vi "PicoScopeospaPowerDetails.vi"(7 "Function":i32, 9 "PICO_USB_POWER_DETAILS In":u8[](array[numeric]), 10 "PICO_USB_POWER_DETAILS Input":T1) -> (1 "PICO_USB_POWER_DETAILS":T1 {"dataPort_"."currentPdo_" format="%x"; "dataPort_"."currentRdo_" format="%x"; "powerport_"."currentPdo_" format="%x"; "powerport_"."currentRdo_" format="%x"}, 2 "PICO_USB_POWER_DETAILS Out":u8[](array[numeric]))   [LabVIEW 2010]
doc: "This is a helper VI to read the C cluster PICO_USB_POWER_DETAILS.\nIt has two functions, controlled via input terminal \"Function\"-\n0 - (default) Outputs U8 array generated from the input cluster.\n1 - Outputs a cluster with data in the from a U8 array input terminal."
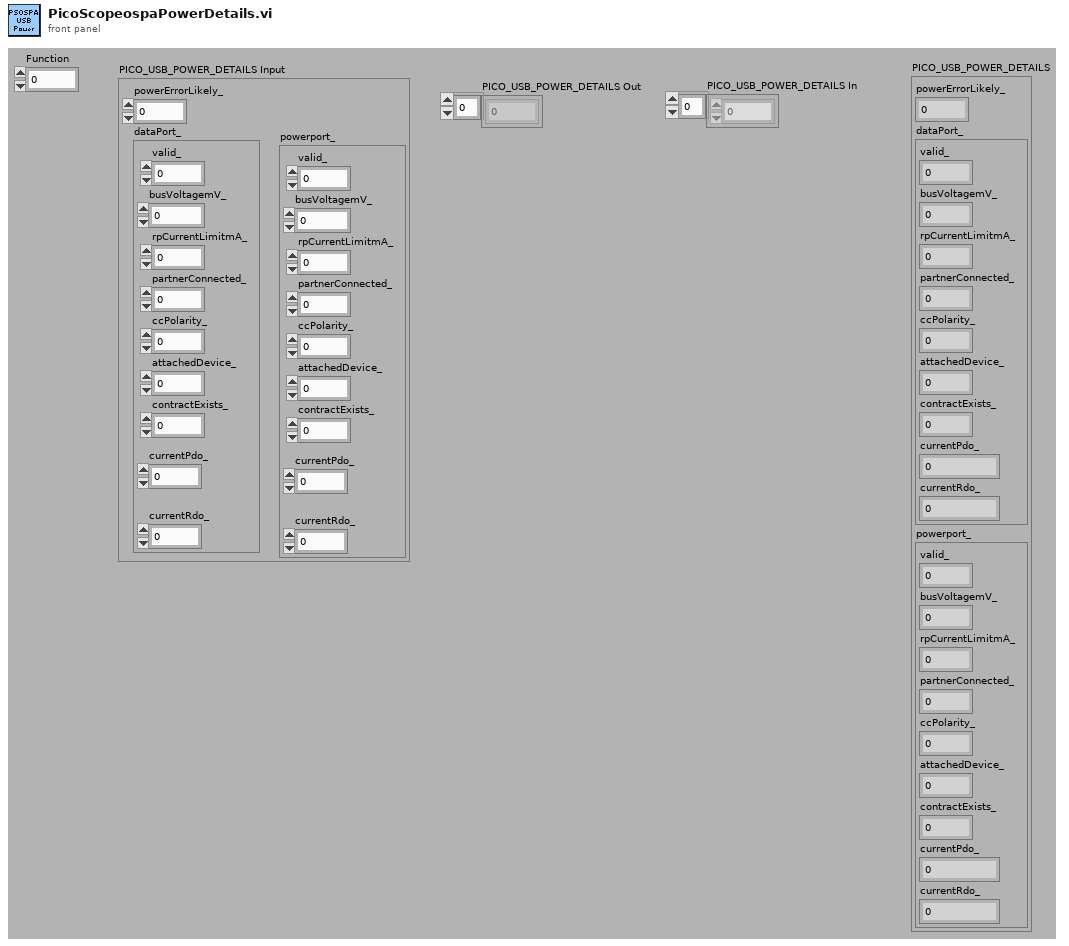
[diagram p1: front panel]
types:
  T1 = cluster{"powerErrorLikely_":u8, "dataPort_":cluster{"valid_":u8, "busVoltagemV_":u32, "rpCurrentLimitmA_":u32, "partnerConnected_":u8, "ccPolarity_":u8, "attachedDevice_":u32, "contractExists_":u8, "currentPdo_":u32, "currentRdo_":u32}, "powerport_":cluster{"valid_":u8, "busVoltagemV_":u32, "rpCurrentLimitmA_":u32, "partnerConnected_":u8, "ccPolarity_":u8, "attachedDevice_":u32, "contractExists_":u8, "currentPdo_":u32, "currentRdo_":u32}}
  T2 = cluster{"valid_":u8, "busVoltagemV_":u32, "rpCurrentLimitmA_":u32, "partnerConnected_":u8, "ccPolarity_":u8, "attachedDevice_":u32, "contractExists_":u8, "currentPdo_":u32, "currentRdo_":u32}
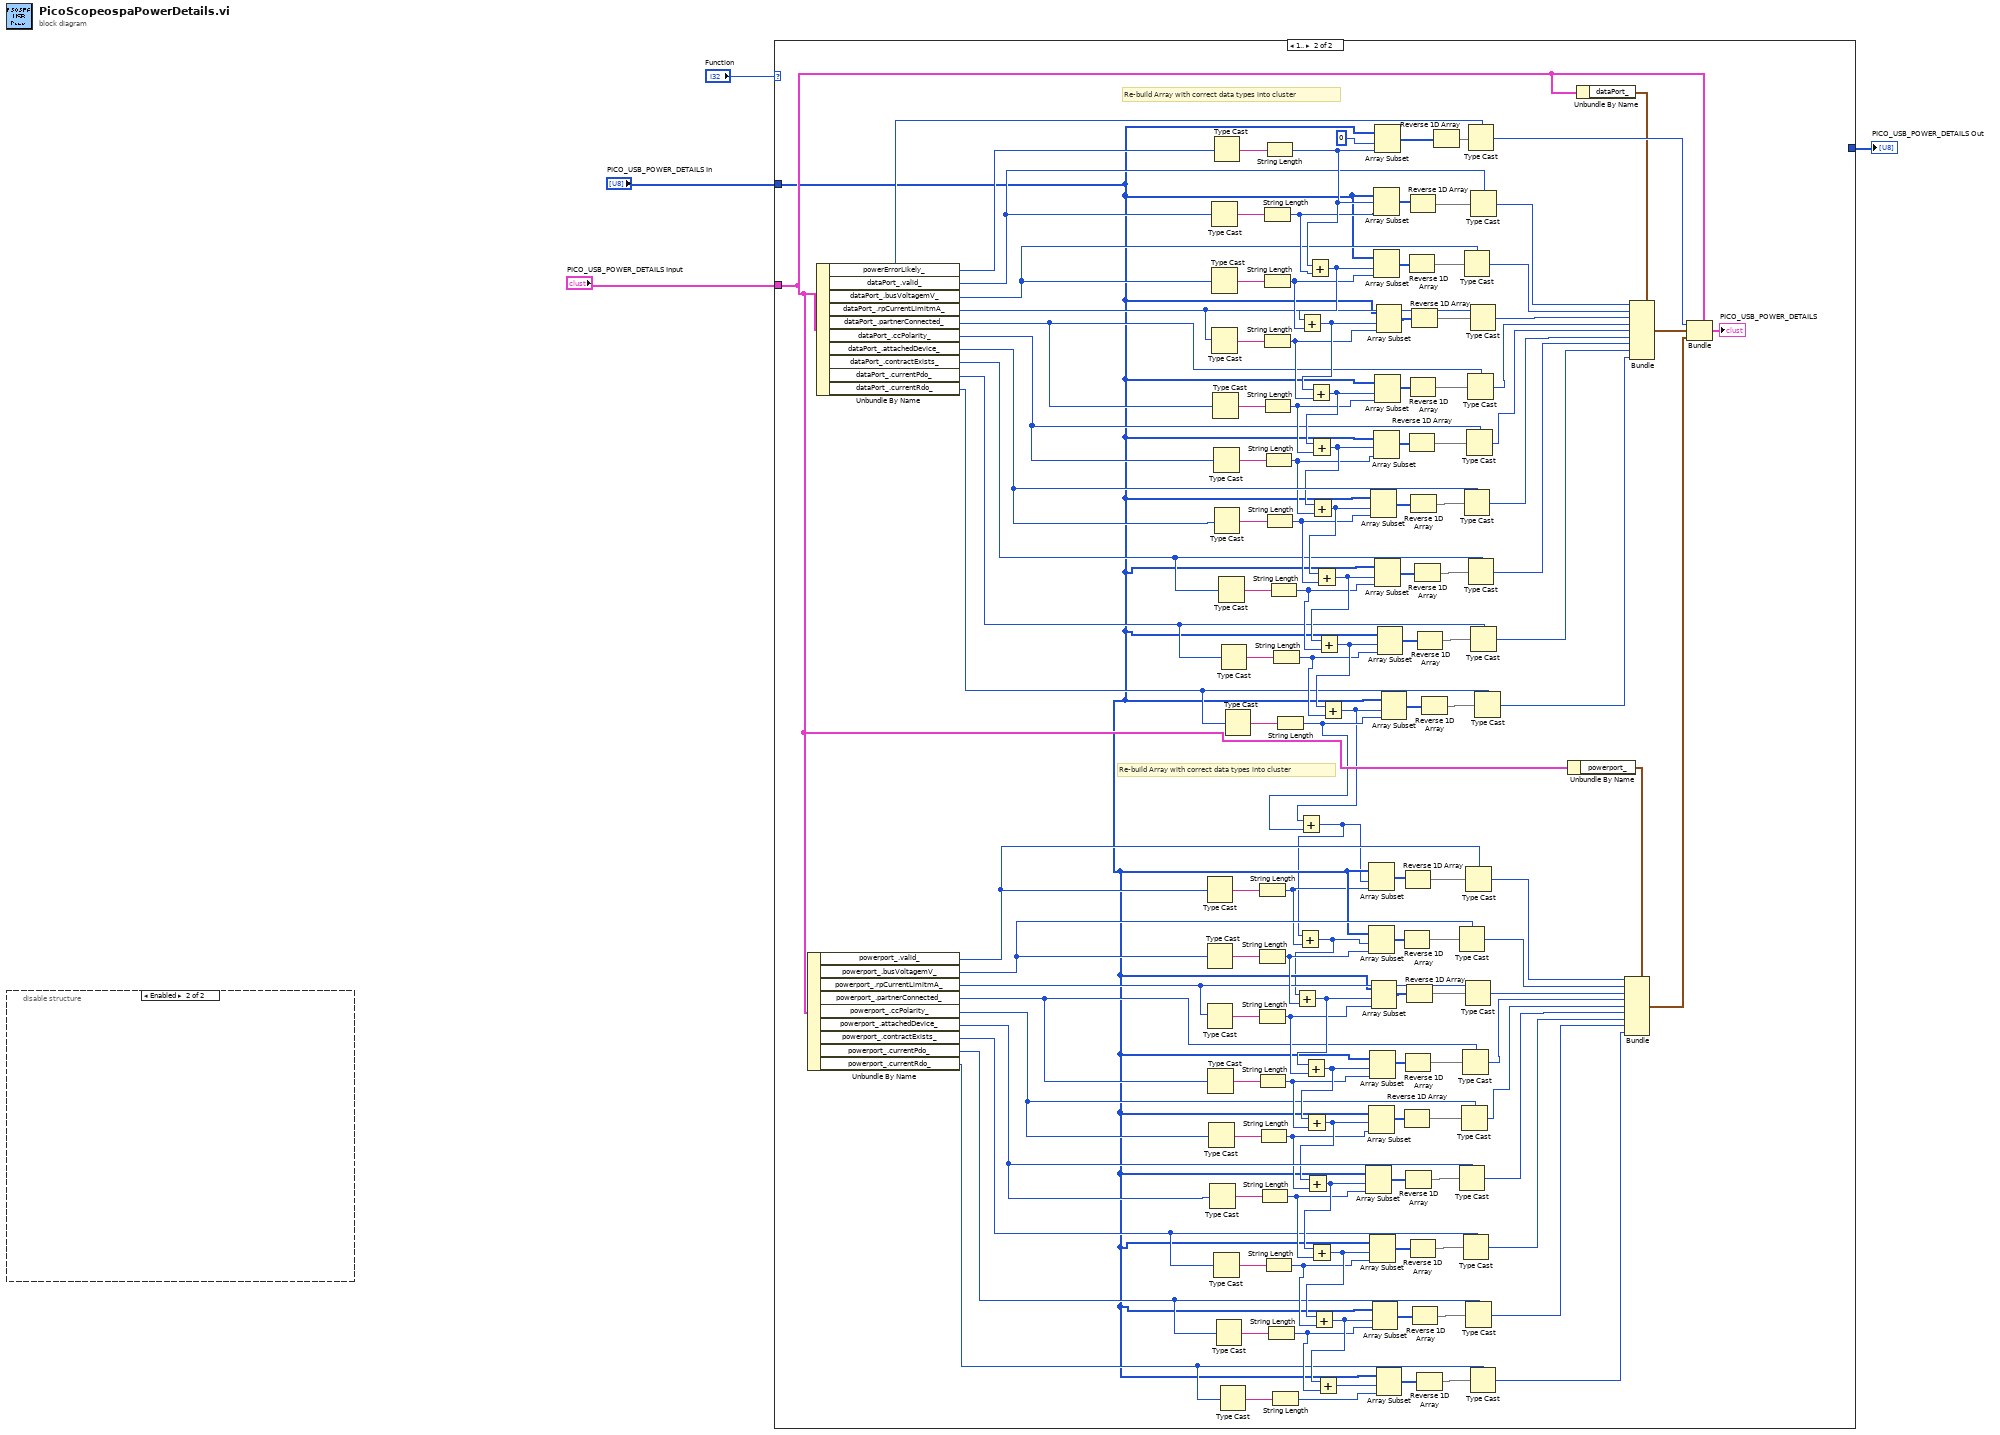
[diagram p0: block diagram]
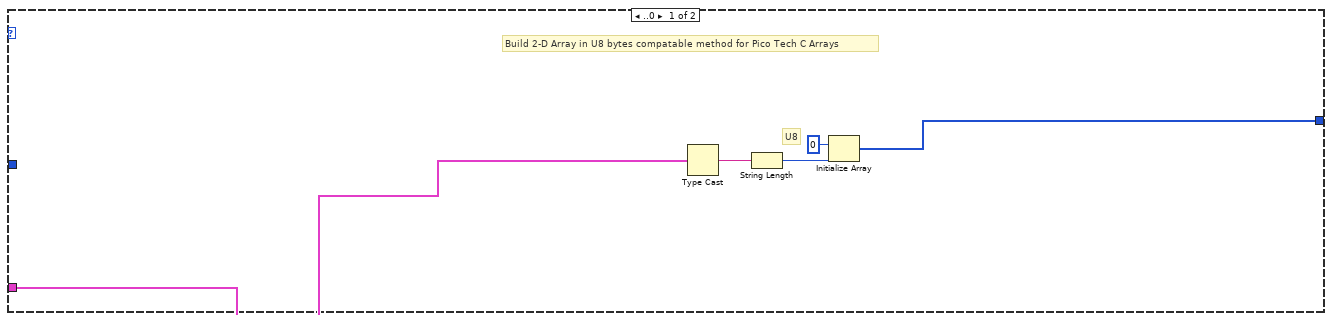
[diagram p2: hidden frame]
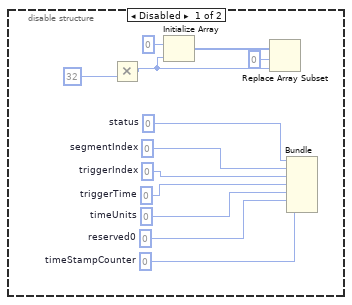
[diagram p3: hidden frame]
diagram:
  n1 = disable-structure shown="Enabled" {
    frame Disabled {
      w12 = u64 0  # timeStampCounter
      w10 = i16 0  # reserved0
      w11 = i16 0  # timeUnits
      w13 = i64 0  # triggerTime
      w14 = u32 0  # triggerIndex
      w15 = u32 0  # segmentIndex
      w16 = u32 0  # status
      n2 = Multiply(y=u32 32) -> (x*y=w8:u32)  [unwired: 1 in]
      n3 = Initialize Array(u8 0 ("element"), w8) -> (w9:u8[])
      n4 = Replace Array Subset(array=w9, new element=w8, index=0) -> ()  [unwired: 1 out]
      n5 = Bundle("status"=w16, "segmentIndex"=w15, "triggerIndex"=w14, "triggerTime"=w13, "timeUnits"=w11, "reserved0"=w10, "timeStampCounter"=w12) -> ()  [unwired: 1 in, 1 out]
    }
    frame Enabled {
    }
  }
  n6 = case shown="1.." "Function" {
    tunnel: "PICO_USB_POWER_DETAILS Input" -> [w18 w29]
    tunnel: [w17 _] -> w2
    tunnel: "PICO_USB_POWER_DETAILS In" -> [_ w27]
    frame ..0 {
      # "U8"
      # "Build 2-D Array in U8 bytes compatable method for Pico Tech C Arrays"
      n7 = Type Cast(x=w18) -> (*(type *) &x=w21:string)  [unwired: 1 in]
      n8 = String Length(string=w21) -> (length=w19:i32)
      n9 = Initialize Array(u8 0 ("element"), w19) -> (w17:u8[])
    }
    frame 1.. {
      # "Re-build Array with correct data types into cluster"
      # "Re-build Array with correct data types into cluster"
      n10 = Unbundle By Name(w29) -> ("powerport_.valid_"=w67:u8, "powerport_.busVoltagemV_"=w63:u32, "powerport_.rpCurrentLimitmA_"=w64:u32, "powerport_.partnerConnected_"=w65:u8, "powerport_.ccPolarity_"=w58:u8, "powerport_.attachedDevice_"=w66:u32, "powerport_.contractExists_"=w32:u8, "powerport_.currentPdo_"=w31:u32, "powerport_.currentRdo_"=w30:u32)
      n11 = Unbundle By Name(w29) -> ("powerErrorLikely_"=w131:u8, "dataPort_.valid_"=w130:u8, "dataPort_.busVoltagemV_"=w126:u32, "dataPort_.rpCurrentLimitmA_"=w127:u32, "dataPort_.partnerConnected_"=w128:u8, "dataPort_.ccPolarity_"=w121:u8, "dataPort_.attachedDevice_"=w129:u32, "dataPort_.contractExists_"=w93:u8, "dataPort_.currentPdo_"=w92:u32, "dataPort_.currentRdo_"=w91:u32)
      n12 = Type Cast(x=w67) -> (*(type *) &x=w79:string)  [unwired: 1 in]
      n13 = Type Cast(x=w63) -> (*(type *) &x=w78:string)  [unwired: 1 in]
      n14 = Type Cast(x=w64) -> (*(type *) &x=w77:string)  [unwired: 1 in]
      n15 = Type Cast(x=w65) -> (*(type *) &x=w76:string)  [unwired: 1 in]
      n16 = Type Cast(x=w58) -> (*(type *) &x=w75:string)  [unwired: 1 in]
      n17 = Type Cast(x=w66) -> (*(type *) &x=w72:string)  [unwired: 1 in]
      n18 = Type Cast(x=w130) -> (*(type *) &x=w147:string)  [unwired: 1 in]
      n19 = Type Cast(x=w126) -> (*(type *) &x=w146:string)  [unwired: 1 in]
      n20 = Type Cast(x=w127) -> (*(type *) &x=w145:string)  [unwired: 1 in]
      n21 = Type Cast(x=w128) -> (*(type *) &x=w144:string)  [unwired: 1 in]
      n22 = Type Cast(x=w121) -> (*(type *) &x=w143:string)  [unwired: 1 in]
      n23 = Type Cast(x=w32) -> (*(type *) &x=w51:string)  [unwired: 1 in]
      n24 = Type Cast(x=w131) -> (*(type *) &x=w148:string)  [unwired: 1 in]
      n25 = Type Cast(x=w129) -> (*(type *) &x=w138:string)  [unwired: 1 in]
      n26 = Type Cast(x=w31) -> (*(type *) &x=w48:string)  [unwired: 1 in]
      n27 = Type Cast(x=w93) -> (*(type *) &x=w110:string)  [unwired: 1 in]
      n28 = Type Cast(x=w30) -> (*(type *) &x=w45:string)  [unwired: 1 in]
      n29 = Type Cast(x=w92) -> (*(type *) &x=w107:string)  [unwired: 1 in]
      n30 = Type Cast(x=w91) -> (*(type *) &x=w104:string)  [unwired: 1 in]
      n31 = String Length(string=w79) -> (length=w26:i32)
      n32 = String Length(string=w78) -> (length=w70:i32)
      n33 = String Length(string=w77) -> (length=w69:i32)
      n34 = String Length(string=w76) -> (length=w68:i32)
      n35 = String Length(string=w75) -> (length=w61:i32)
      n36 = String Length(string=w72) -> (length=w38:i32)
      n37 = String Length(string=w147) -> (length=w136:i32)
      n38 = String Length(string=w146) -> (length=w134:i32)
      n39 = String Length(string=w145) -> (length=w133:i32)
      n40 = String Length(string=w144) -> (length=w132:i32)
      n41 = String Length(string=w143) -> (length=w124:i32)
      n42 = String Length(string=w51) -> (length=w37:i32)
      n43 = String Length(string=w148) -> (length=w139:i32)
      n44 = String Length(string=w138) -> (length=w99:i32)
      n45 = String Length(string=w48) -> (length=w36:i32)
      n46 = String Length(string=w110) -> (length=w98:i32)
      n47 = String Length(string=w45) -> (length=w43:i32)
      n48 = String Length(string=w107) -> (length=w97:i32)
      n49 = String Length(string=w104) -> (length=w23:i32)
      n50 = Add(x=w139, y=w136) -> (x+y=w135:i32)
      n51 = Add(x=w135, y=w134) -> (x+y=w142:i32)
      n52 = Add(x=w142, y=w133) -> (x+y=w141:i32)
      n53 = Add(x=w141, y=w132) -> (x+y=w125:i32)
      n54 = Add(x=w125, y=w124) -> (x+y=w102:i32)
      n55 = Add(x=w102, y=w99) -> (x+y=w101:i32)
      n56 = Add(x=w101, y=w98) -> (x+y=w100:i32)
      n57 = Add(x=w100, y=w97) -> (x+y=w22:i32)
      n58 = Add(x=w22, y=w23) -> (x+y=w24:i32)
      n59 = Add(x=w24, y=w26) -> (x+y=w25:i32)
      n60 = Add(x=w25, y=w70) -> (x+y=w74:i32)
      n61 = Add(x=w74, y=w69) -> (x+y=w73:i32)
      n62 = Add(x=w73, y=w68) -> (x+y=w62:i32)
      n63 = Add(x=w62, y=w61) -> (x+y=w41:i32)
      n64 = Add(x=w41, y=w38) -> (x+y=w40:i32)
      n65 = Add(x=w40, y=w37) -> (x+y=w39:i32)
      n66 = Add(x=w39, y=w36) -> (x+y=w44:i32)
      n67 = Array Subset(array=w27, index=w41, length=w38) -> (w71:u8[])
      n68 = Array Subset(array=w27, index=w24, length=w26) -> (w88:u8[])
      n69 = Array Subset(array=w27, index=w25, length=w70) -> (w85:u8[])
      n70 = Array Subset(array=w27, index=w62, length=w61) -> (w59:u8[])
      n71 = Array Subset(array=w27, index=w73, length=w68) -> (w82:u8[])
      n72 = Array Subset(array=w27, index=w40, length=w37) -> (w50:u8[])
      n73 = Array Subset(array=w27, index=w102, length=w99) -> (w137:u8[])
      n74 = Array Subset(array=w27, index=w74, length=w69) -> (w84:u8[])
      n75 = Array Subset(array=w27, index=w39, length=w36) -> (w47:u8[])
      n76 = Array Subset(array=w27, index=w139, length=w136) -> (w158:u8[])
      n77 = Array Subset(array=w27, index=w135, length=w134) -> (w154:u8[])
      n78 = Array Subset(array=w27, index=w125, length=w124) -> (w122:u8[])
      n79 = Array Subset(array=w27, index=u8 0, length=w139) -> (w118:u8[])
      n80 = Array Subset(array=w27, index=w141, length=w132) -> (w151:u8[])
      n81 = Array Subset(array=w27, index=w101, length=w98) -> (w109:u8[])
      n82 = Array Subset(array=w27, index=w142, length=w133) -> (w153:u8[])
      n83 = Array Subset(array=w27, index=w44, length=w43) -> (w42:u8[])
      n84 = Array Subset(array=w27, index=w100, length=w97) -> (w106:u8[])
      n85 = Array Subset(array=w27, index=w22, length=w23) -> (w103:u8[])
      n86 = Reverse 1D Array(array=w85) -> (reversed array=w86:u8[])
      n87 = Reverse 1D Array(array=w59) -> (reversed array=w60:u8[])
      n88 = Reverse 1D Array(array=w88) -> (reversed array=w87:u8[])
      n89 = Reverse 1D Array(array=w82) -> (reversed array=w81:u8[])
      n90 = Reverse 1D Array(array=w71) -> (reversed array=w80:u8[])
      n91 = Reverse 1D Array(array=w84) -> (reversed array=w83:u8[])
      n92 = Reverse 1D Array(array=w154) -> (reversed array=w155:u8[])
      n93 = Reverse 1D Array(array=w122) -> (reversed array=w123:u8[])
      n94 = Reverse 1D Array(array=w158) -> (reversed array=w157:u8[])
      n95 = Reverse 1D Array(array=w151) -> (reversed array=w150:u8[])
      n96 = Reverse 1D Array(array=w50) -> (reversed array=w52:u8[])
      n97 = Reverse 1D Array(array=w137) -> (reversed array=w149:u8[])
      n98 = Reverse 1D Array(array=w153) -> (reversed array=w152:u8[])
      n99 = Reverse 1D Array(array=w47) -> (reversed array=w49:u8[])
      n100 = Reverse 1D Array(array=w109) -> (reversed array=w111:u8[])
      n101 = Reverse 1D Array(array=w42) -> (reversed array=w46:u8[])
      n102 = Reverse 1D Array(array=w106) -> (reversed array=w108:u8[])
      n103 = Reverse 1D Array(array=w103) -> (reversed array=w105:u8[])
      n104 = Reverse 1D Array(array=w118) -> (reversed array=w156:u8[])
      n105 = Type Cast(type=w63, x=w86) -> (*(type *) &x=w54:u32)
      n106 = Type Cast(type=w66, x=w80) -> (*(type *) &x=w56:u32)
      n107 = Type Cast(type=w58, x=w60) -> (*(type *) &x=w57:u8)
      n108 = Type Cast(type=w65, x=w81) -> (*(type *) &x=w89:u8)
      n109 = Type Cast(type=w32, x=w52) -> (*(type *) &x=w35:u8)
      n110 = Type Cast(type=w126, x=w155) -> (*(type *) &x=w116:u32)
      n111 = Type Cast(type=w129, x=w149) -> (*(type *) &x=w119:u32)
      n112 = Type Cast(type=w64, x=w83) -> (*(type *) &x=w90:u32)
      n113 = Type Cast(type=w67, x=w87) -> (*(type *) &x=w55:u8)
      n114 = Type Cast(type=w31, x=w49) -> (*(type *) &x=w34:u32)
      n115 = Type Cast(type=w121, x=w123) -> (*(type *) &x=w120:u8)
      n116 = Type Cast(type=w128, x=w150) -> (*(type *) &x=w159:u8)
      n117 = Type Cast(type=w131, x=w156) -> (*(type *) &x=w115:u8)
      n118 = Type Cast(type=w93, x=w111) -> (*(type *) &x=w96:u8)
      n119 = Type Cast(type=w127, x=w152) -> (*(type *) &x=w160:u32)
      n120 = Type Cast(type=w30, x=w46) -> (*(type *) &x=w33:u32)
      n121 = Type Cast(type=w130, x=w157) -> (*(type *) &x=w117:u8)
      n122 = Type Cast(type=w92, x=w108) -> (*(type *) &x=w95:u32)
      n123 = Type Cast(type=w91, x=w105) -> (*(type *) &x=w94:u32)
      n124 = Unbundle By Name(w29) -> ("powerport_"=w53:T2)
      n125 = Unbundle By Name(w29) -> ("dataPort_"=w113:T2)
      n126 = Bundle(cluster=w53, "valid_"=w55, "busVoltagemV_"=w54, "rpCurrentLimitmA_"=w90, "partnerConnected_"=w89, "ccPolarity_"=w57, "attachedDevice_"=w56, "contractExists_"=w35, "currentPdo_"=w34, "currentRdo_"=w33) -> (w28:T2)
      n127 = Bundle(cluster=w113, "valid_"=w117, "busVoltagemV_"=w116, "rpCurrentLimitmA_"=w160, "partnerConnected_"=w159, "ccPolarity_"=w120, "attachedDevice_"=w119, "contractExists_"=w96, "currentPdo_"=w95, "currentRdo_"=w94) -> (w112:T2)
      n128 = Bundle(cluster=w29, "powerErrorLikely_"=w115, "dataPort_"=w112, "powerport_"=w28) -> (→"PICO_USB_POWER_DETAILS":T1)
    }
  }
  "PICO_USB_POWER_DETAILS Out" <- w2
